vi "Sep axes ini result in order.vi"(2 "Sep. axes to initialize":string[](array[string])=["B"], 3 "Sep. axes initialized?":bool[](array[boolean])) -> (14 "A/B initialized?`":bool[](array[boolean]))   [LabVIEW 2026]
doc: "Returns result of Sep. axes initialized? according to order of Sep. axes to initialize."
panel:
  # "Returns result of \"Sep. axes initialized?\"\naccording to order of \"Sep. axes to initialize\"."
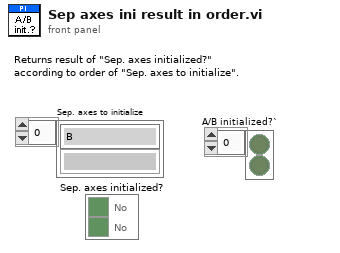
[diagram p1: front panel]
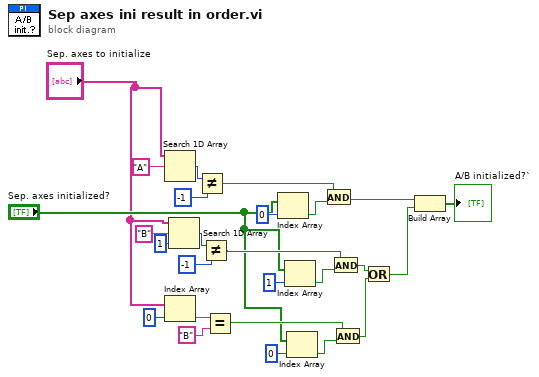
[diagram p0: block diagram]
diagram:
  n1 = Search 1D Array(1D array="Sep. axes to initialize", element="A" ("String")) -> (index of element=w25:i32)  [unwired: 1 out]
  n2 = Index Array(array="Sep. axes to initialize", index=0) -> (element=w10:string)
  n3 = Search 1D Array(1D array="Sep. axes to initialize", element="B" ("String"), start index (0)=1) -> (index of element=w22:i32)
  n4 = Not Equal?(x=w25, y=-1) -> (x != y?=w19:bool)
  n5 = Not Equal?(x=w22, y=-1) -> (x != y?=w13:bool)
  n6 = Equal?(x=w10, y="B" ("String")) -> (x = y?=w6:bool)
  n7 = Index Array(array="Sep. axes initialized?", index=0) -> (element=w18:bool)
  n8 = Index Array(array="Sep. axes initialized?", index=1) -> (element=w15:bool)
  n9 = Index Array(array="Sep. axes initialized?", index=0) -> (element=w8:bool)
  n10 = And(x=w19, y=w18) -> (x .and. y?=w16:bool)
  n11 = And(x=w13, y=w15) -> (x .and. y?=w12:bool)
  n12 = And(x=w6, y=w8) -> (x .and. y?=w4:bool)
  n13 = Or(x=w12, y=w4) -> (x .or. y?=w3:bool)
  n14 = Build Array(w16, w3) -> (→"A/B initialized?`":bool[])
